vi "Test_SendAndAskForReply.vi"(8 "error in (no error)":errorcluster) -> (0 "error out":errorcluster)   [LabVIEW 2020, in "horiba.test.lvlib"]
uses:
  horiba.test.lvlib
  <vilib>/addons/_JKI Toolkits/Caraya/classes/Assert/Assert Not Error.vi
  Classes/Communicator/Communicator.lvclass
  6eb843e0-10d8-45cd-a1eb-a4d1fb80ef5a.vi
  <vilib>/addons/_JKI Toolkits/Caraya/classes/Assert/Assert True.vi
panel:
  # "Connector Pane"
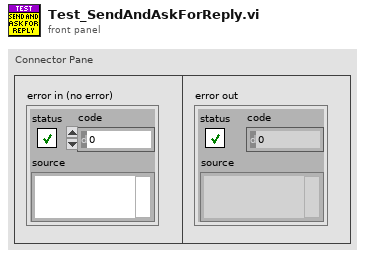
[diagram p1: front panel]
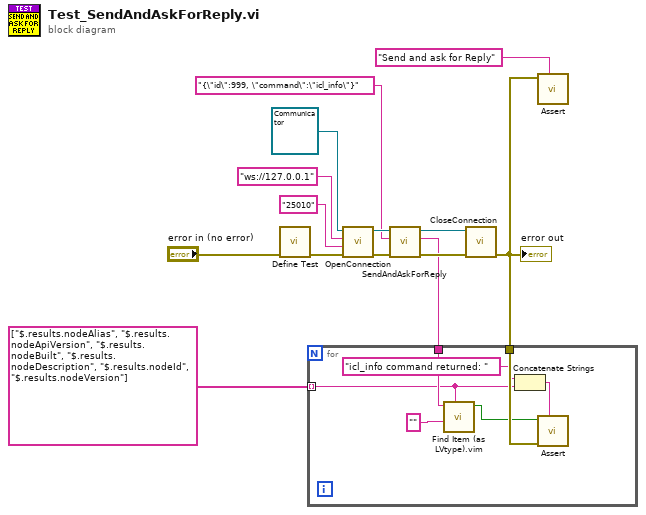
[diagram p0: block diagram]
diagram:
  n1 = call <vilib>:"Define Test.vi"("error in (no error)"="error in (no error)") -> ("error out"=w11:errorcluster)  [unwired: 9 in, 1 out]
  n2 = call-dynamic "OpenConnection.vi"("error in (no error)"=w11, "WS Server Port"="25010", "WS Server IP"="ws://127.0.0.1", "Communicator in"=refnum<class "Communicator.lvclass"> refnum) -> ("error out"=w8:errorcluster, "Communicator out"=w7:refnum<class "Communicator.lvclass">)  [unwired: 5 in, 1 out]
  n3 = call-dynamic "SendAndAskForReply.vi"("error in (no error)"=w8, "String to be sent"="{\"id\":999, \"command\":\"icl_info\"}" ("send command"), "Communicator in"=w7) -> ("error out"=w6:errorcluster, "Data"=w2:string, "Communicator out"=w5:refnum<class "Communicator.lvclass">)  [unwired: 6 in]
  n4 = call-dynamic "CloseConnection.vi"("error in (no error)"=w6, "Communicator in"=w5) -> ("error out"=w4:errorcluster)  [unwired: 8 in, 1 out]
  "error out" <- w4
  n5 = for {
    tunnel: w4 -> [w21]
    tunnel: w2 -> [w18]
    tunnel: string[] ["$.results.nodeAlias", "$.results.nodeApiVersion", "$.results.nodeBuilt", "$.results.nodeDescription", "$.results.nodeId", "$.results.nodeVersion"] -> [w17] mode=indexing
    n6 = call "Find Item (as LVtype).vim"("$Path or Item Name"=w17, "Data Type and Default Value"="", "JSON"=w18) -> ("Found"=w20:bool)  [unwired: 5 in, 3 out]
    n7 = Concatenate Strings("icl_info command returned: " ("Label"), w17) -> (w16:string)
    n8 = call-poly <vilib>:"Assert.vi"("Label"=w16, "error in (no error)"=w21, "True?"=w20) -> ()  [unwired: 7 in, 2 out]
  }
  n9 = call-poly <vilib>:"Assert.vi"("Label"="Send and ask for Reply", "Not Error?"=w4) -> ()  [unwired: 8 in, 2 out]
